vi "Write Control.vi"(8 "error in":errorcluster, 10 "Producer Control":T1, 11 "Chiller Cluster - 2 Channel.lvclass":refnum<class "Climate Chamber - 2 Channel.lvclass">) -> (0 "error out":errorcluster, 3 "output cluster":refnum<class "Climate Chamber - 2 Channel.lvclass">)   [LabVIEW 2023, in "Climate Chamber - 2 Channel.lvclass"]
uses:
  Climate Chamber - 2 Channel.lvclass
  Climate Chamber - 2 Channel.lvclass/Climate Chamber - 2 Channel.ctl
  36f3130d-3290-4452-ba15-24beea2e5298.vi
  36f3130d-3290-4452-ba15-24beea2e5298.vi/4bc1c15b-36ab-481f-b8dd-c64075ce723a.vi
  36f3130d-3290-4452-ba15-24beea2e5298.vi/d83cb72b-7713-41fc-a3d1-682de79cf574.vi
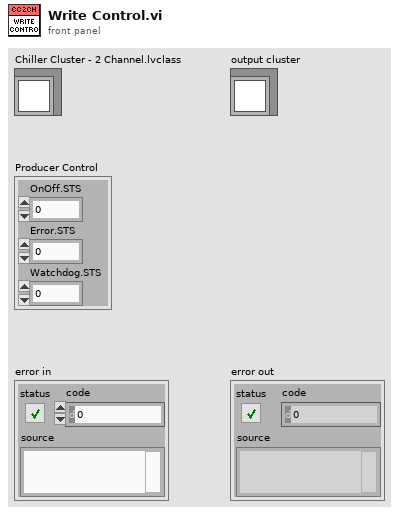
[diagram p1: front panel]
types:
  T1 = cluster{"OnOff.STS":i32, "Error.STS":i32, "Watchdog.STS":i32}
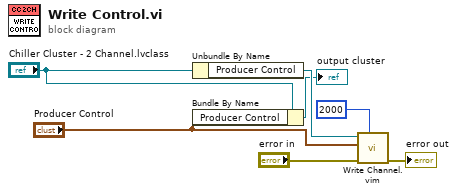
[diagram p0: block diagram]
diagram:
  n1 = Unbundle By Name("Chiller Cluster - 2 Channel.lvclass") -> ("Producer Control"=w3:refnum<k21>)
  n2 = Bundle By Name(cluster="Chiller Cluster - 2 Channel.lvclass", "Producer Control"="Producer Control") -> (→"output cluster":refnum<class "Climate Chamber - 2 Channel.lvclass">)
  n3 = call "Write Channel.vim"("Timeout (ms)"=2000, "error in"="error in", "Data in"="Producer Control", "ADAS HIL Channel in"=w3) -> ("error out"=→"error out":errorcluster)  [unwired: 5 in, 2 out]
